vi "layer_switch.vi"() -> ()   [LabVIEW 2020]
panel:
  out "Array":dbl[](array[numeric])
  in  "channel 15":bool
  in  "channel 14":bool
  in  "channel 13":bool
  in  "channel 12":bool
  in  "channel 11":bool
  in  "channel 10":bool
  in  "channel 9":bool
  in  "channel 8":bool
  in  "channel 7":bool
  in  "channel 6":bool
  in  "channel 5":bool
  in  "channel 4":bool
  in  "channel 3":bool
  in  "channel 2":bool
  in  "channel 1":bool
  in  "channel 0":bool
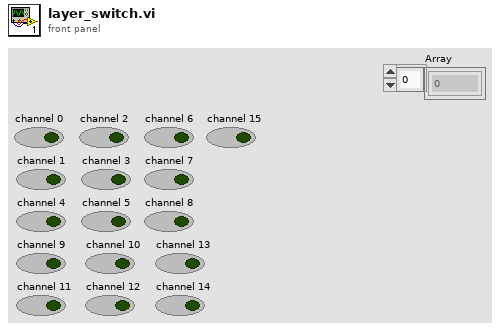
[diagram p1: front panel]
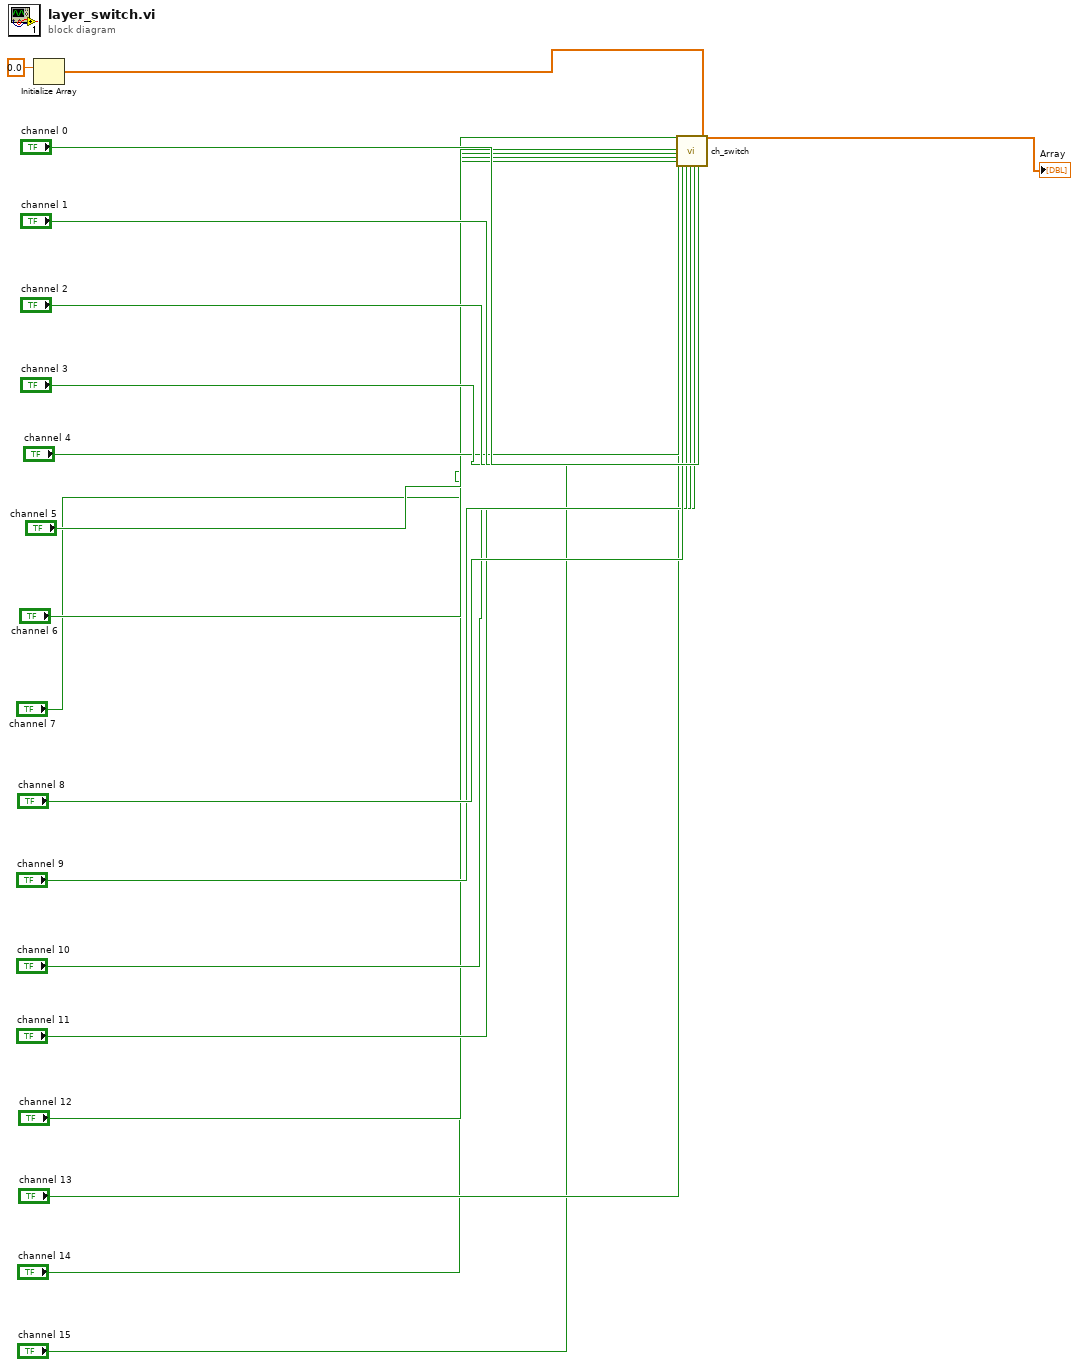
[diagram p0: block diagram]
diagram:
  n1 = Initialize Array(0.0 ("element")) -> (w2:dbl[])  [unwired: 1 in]
  n2 = call "ch_switch.vi"("channel 14"="channel 14", "channel 4"="channel 4", "channel 13"="channel 13", "channel 5"="channel 5", "channel 12"="channel 12", "channel 6"="channel 6", "channel 7"="channel 7", "channel 3"="channel 3", "channel 8"="channel 8", "channel 15"="channel 15", "channel 9"="channel 9", "channel 2"="channel 2", "channel 10"="channel 10", "channel 1"="channel 1", "channel 11"="channel 11", "channel 0"="channel 0", "Array in"=w2) -> ("Array out"=→"Array":dbl[])  [unwired: 10 in]
